vi "Pre Launch Init.vi"(11 "Main View in":refnum<class "Main View.lvclass">) -> (0 "error out":errorcluster, 3 "Main View out":refnum<class "Main View.lvclass">)   [LabVIEW 2013, in "Main View.lvlib" / "Main View.lvclass"]
doc: "(<B>Filename</B>: Actor Framework.lvlib:Actor.lvclass:Pre Launch Init.vi)\n\nDefines behavior that occurs after the Launch Actor method is invoked but before the actor's Actor Core method begins running.\n\nThe Pre Launch Init method is guaranteed to finish before the Launch Actor method returns to its caller and before the actor itself receives any messages. Any references that the Pre Launch Init method obtains are guaranteed to have the same lifetime as the actor itself. Any errors that the Pre Launch Init method returns will abort the launch.\n\nBy default, this method does nothing. A descendant class may override it to define behavior."
uses:
  Main View.lvclass
  Main View.lvclass/Main View.ctl
  <vilib>/ActorFrameworkMVC/View Actor/View Actor.lvclass
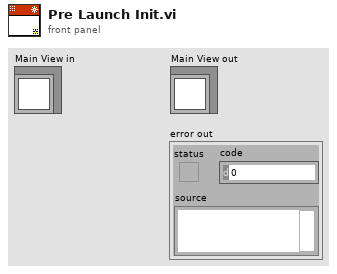
[diagram p1: front panel]
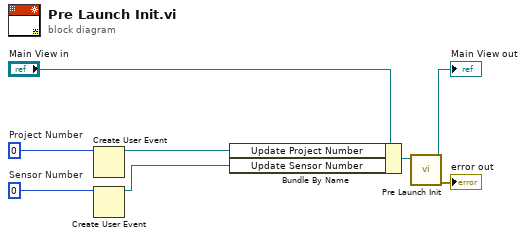
[diagram p0: block diagram]
diagram:
  w2 = 0  # Sensor Number
  w3 = 0  # Project Number
  n1 = Create User Event(user event datatype=w3) -> (user event=w5:refnum<user-event>)  [unwired: 1 in, 1 out]
  n2 = Create User Event(user event datatype=w2) -> (user event=w1:refnum<user-event>)  [unwired: 1 in, 1 out]
  n3 = Bundle By Name(cluster="Main View in", "Update Project Number"=w5, "Update Sensor Number"=w1) -> (w6:refnum<class "Main View.lvclass">)
  n4 = call-parent "Pre Launch Init.vi"("Actor in"=w6) -> ("error out"=→"error out":errorcluster, "Actor out"=→"Main View out":refnum<class "Main View.lvclass">)  [unwired: 9 in]
